vi "GD_Check_All .vi"(8 "error in (no error)":errorcluster, 11 "DBlink":string="Driver={ODBC Driver 17 for SQL Server};Server=localhost\\SQLEXPRESS;Database=ZDX201;UID=labview;PWD=Dsa@54137926") -> (0 "error out":errorcluster, 2 "資料是否完整":i32)   [LabVIEW 2019]
uses:
  <vilib>/addons/database/Connection.llb/DB Tools Open Connec (String).vi
  <vilib>/addons/database/Connection.llb/Conn Execute.vi
  <vilib>/addons/database/Recordset.llb/Rec Fetch Recordset Data (R).vi
  <vilib>/addons/database/Recordset.llb/Rec Destroy - Connection.vi
  <vilib>/addons/database/_DB Variant To Data/Database Variant To Data.xnode
  <vilib>/addons/database/NI_Database_API.lvlib
panel:
  out "查詢結果":string="SELECT \n       [barcode A]\n      ,[barcode B]\n  FROM [ZDX201].[dbo].[workplace_data]\n  where [workplace_name_id]>9 and [workplace_name_id]<11 and ([barcode A] is not null or [barcode B] is not null)\n  order by [workplace_name_id]"
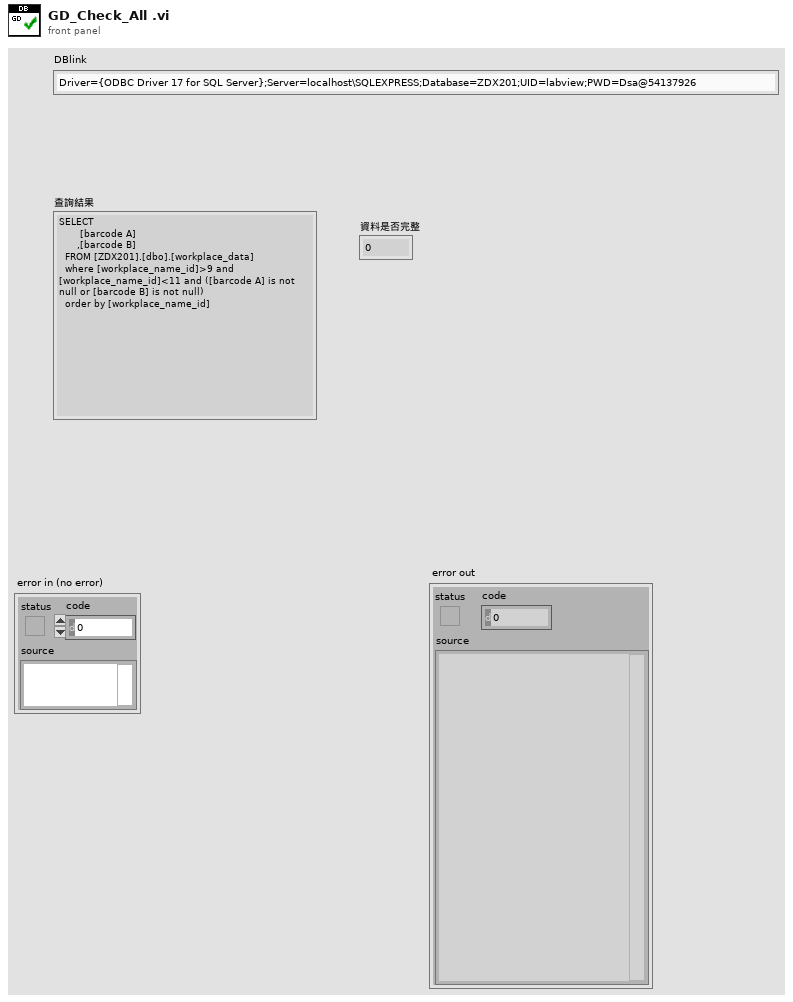
[diagram p1: front panel]
types:
  T1 = typedef "NI_Database_API.lvlib/Conn ObjectReference.ctl" = refnum<k1>
  T2 = typedef "NI_Database_API.lvlib/Rec ObjectReference.ctl" = refnum<k1>
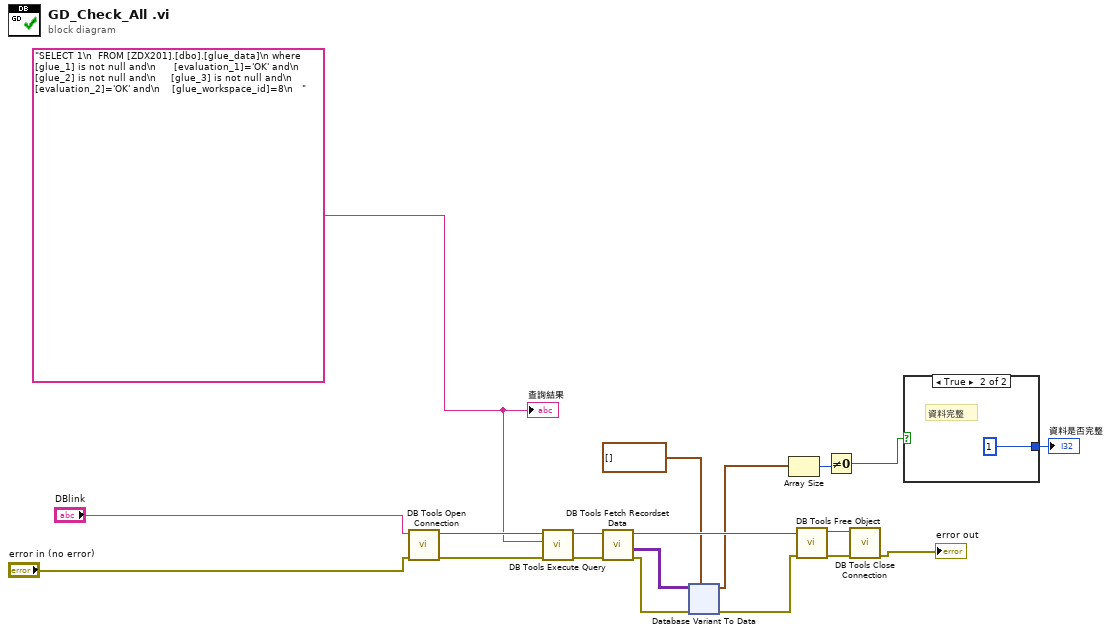
[diagram p0: block diagram]
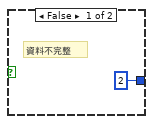
[diagram p2: hidden frame]
diagram:
  w3 = "SELECT 1\n  FROM [ZDX201].[dbo].[glue_data]\n where  [glue_1] is not null and\n      [evaluation_1]='OK' and\n      [glue_2] is not null and\n     [glue_3] is not null and\n    [evaluation_2]='OK' and\n    [glue_workspace_id]=8\n   "
  n1 = call-poly <vilib>:"DB Tools Open Connection.vi"("error in (no error)"="error in (no error)", "connection information"="DBlink") -> ("error out"=w19:errorcluster, "connection reference"=w18:T1)  [unwired: 6 in]
  n2 = call-poly <vilib>:"DB Tools Execute Query.vi"("error in (no error)"=w19, "SQL query"=w3, "connection reference"=w18) -> ("error out"=w16:errorcluster, "recordset reference"=w17:T2)  [unwired: 5 in]
  n3 = call-poly <vilib>:"DB Tools Fetch Recordset Data.vi"("error in (no error)"=w16, "recordset reference"=w17) -> ("error out"=w11:errorcluster, "recordset data"=w10:variant[][], "recordset reference out"=w12:T2)  [unwired: 3 in]
  n4 = xnode "Database Variant To Data"("database variant"=w10, "error in (no error)"=w11, "type"=cluster{i32}[] [] ("Workplace: assemble")) -> ("data"=w7:cluster{i32}[], "error out"=w13:errorcluster)
  n5 = Array Size(array=w7) -> (size(s)=w8:i32)
  n6 = call-poly <vilib>:"DB Tools Free Object.vi"("error in (no error)"=w13, "recordset reference"=w12) -> ("error out"=w14:errorcluster, "connection reference"=w15:T1)  [unwired: 8 in]
  n7 = Not Equal To 0?(x=w8) -> (x != 0?=w6:bool)
  n8 = call <vilib>:"DB Tools Close Connection.vi"("error in (no error)"=w14, "connection reference"=w15) -> ("error out"=→"error out":errorcluster)  [unwired: 5 in]
  n9 = case shown="True" w6 {
    tunnel: [2 1] -> w1
    frame False {
      # "資料不完整"
    }
    frame True {
      # "資料完整"
    }
  }
  "資料是否完整" <- w1
  "查詢結果" <- w3
